vi "RTS Toggle Complete Buttons.vi"(7 "Delay":bool, 8 "Error In":errorcluster, 9 "Door Open Sequence:":T5, 10 "Times Up?":bool, 11 "Station 1-8 Data in in":T1 {"Station Slide"."Chamber 1-1"."Start Time" format="%<%X\n%x>T"; "Station Slide"."Chamber 1-1"."End Time" format="%<%X\n%x>T"; "Station Slide"."Time Count (s)" format="%.2f"; "Station Cab"."Chamber 1-1"."Start Time" format="%<%X\n%x>T"; "Station Cab"."Chamber 1-1"."End Time" format="%<%X\n%x>T"; "Station Cab"."Time Count (s)" format="%.2f"; "Station Freezer"."Chamber 1-1"."Start Time" format="%<%X\n%x>T"; "Station Freezer"."Chamber 1-1"."End Time" format="%<%X\n%x>T"; "Station Freezer"."Time Count (s)" format="%.2f"}) -> (0 "Error Out":errorcluster, 3 "Station 1-8 Data in out":T1 {"Station Slide"."Chamber 1-1"."Start Time" format="%<%X\n%x>T"; "Station Slide"."Chamber 1-1"."End Time" format="%<%X\n%x>T"; "Station Slide"."Time Count (s)" format="%.2f"; "Station Cab"."Chamber 1-1"."Start Time" format="%<%X\n%x>T"; "Station Cab"."Chamber 1-1"."End Time" format="%<%X\n%x>T"; "Station Cab"."Time Count (s)" format="%.2f"; "Station Freezer"."Chamber 1-1"."Start Time" format="%<%X\n%x>T"; "Station Freezer"."Chamber 1-1"."End Time" format="%<%X\n%x>T"; "Station Freezer"."Time Count (s)" format="%.2f"})   [LabVIEW 2016]
uses:
  Type Definitions/RTS Door Ops Sequence.ctl
  Type Definitions/RTS Station Relay Ops.ctl
  Type Definitions/RTS Door Opener Indicator.ctl
  Type Definitions/RTS Door Ops Client.ctl
  Type Definitions/RTS Door Opening Schedule.ctl
panel:
  # "Chamber Conditions:"
  # "Chamber Conditions:"
  # "Chamber Conditions:"
  # "Chamber Conditions:"
  # "Chamber Conditions:"
  # "Chamber Conditions:"
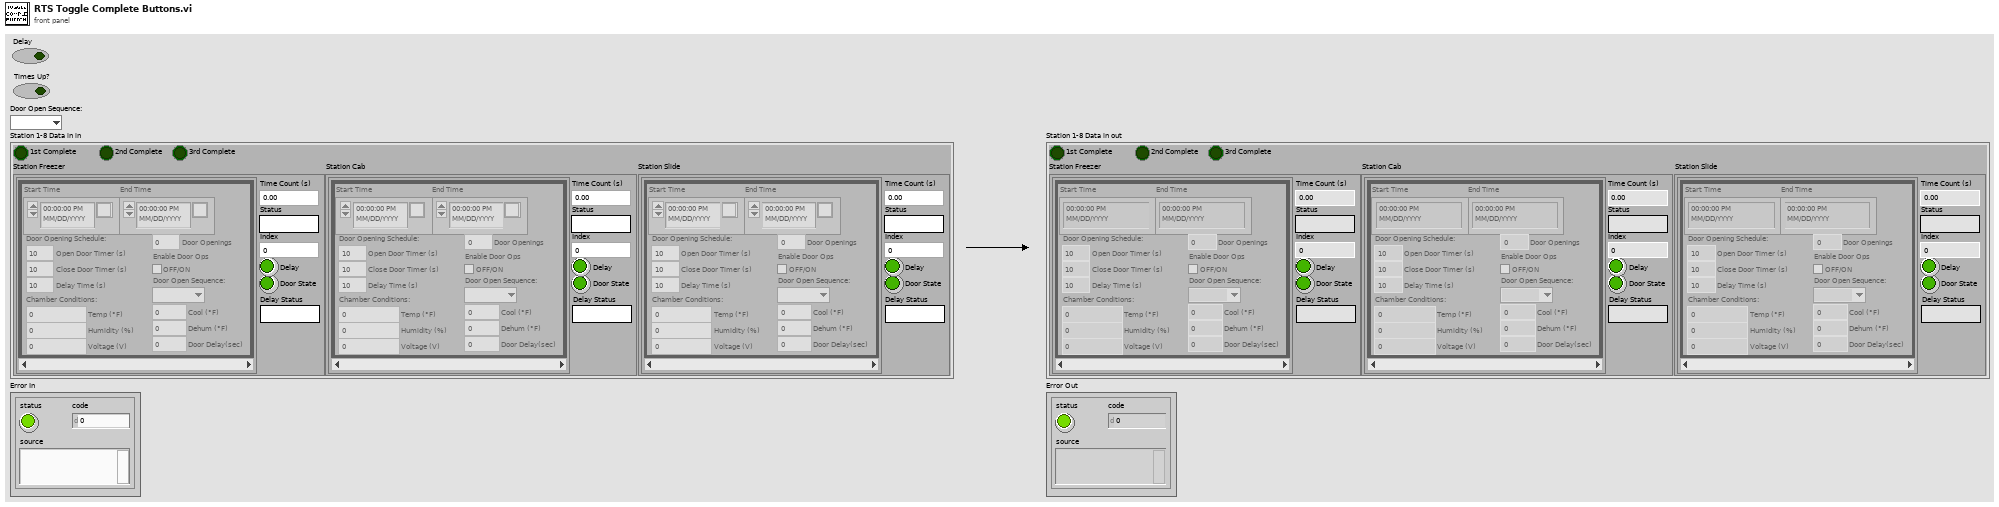
[diagram p1: front panel]
types:
  T1 = typedef "RTS Station Relay Ops.ctl" = cluster{"Station Freezer":T2, "Station Cab":T2, "Station Slide":T2, "1st Complete":bool, "2nd Complete":bool, "3rd Complete":bool}
  T2 = typedef "RTS Door Opener Indicator.ctl" = cluster{"Time Count (s)":dbl, "Status":string, "Door State":bool, "Delay":bool, "Chamber 1-1":T3[], "Index":i32, "Delay Status":string}
  T3 = typedef "RTS Door Ops Client.ctl" = cluster{"End Time":timestamp, "Start Time":timestamp, "Door Opening Schedule:":T4, "Enable Door Ops":bool, "Door Openings":u32, "Temp (°F)":dbl, "Humidity (%)":dbl, "Voltage (V)":dbl, "Door Open Sequence:":T5, "Door Delay(sec)":dbl, "Dehum (°F)":dbl, "Cool (°F)":dbl}
  T4 = typedef "RTS Door Opening Schedule.ctl" = cluster{"Open Door Timer (s)":dbl, "Delay Time (s)":dbl, "Close Door Timer (s)":dbl}
  T5 = typedef "RTS Door Ops Sequence.ctl" = enum16{"", "1st", "2nd", "3rd"}
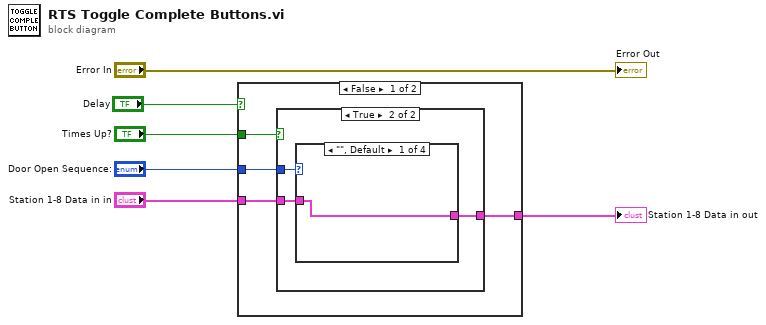
[diagram p0: block diagram]
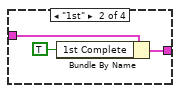
[diagram p3: hidden frame]
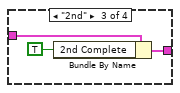
[diagram p4: hidden frame]
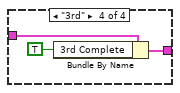
[diagram p5: hidden frame]
diagram:
  n1 = case shown="False" "Delay" {
    tunnel: "Door Open Sequence:" -> [w10 _]
    tunnel: "Station 1-8 Data in in" -> [w9 w25]
    tunnel: "Times Up?" -> [w8 _]
    tunnel: [w7 w25] -> w3
    frame False {
      n2 = case shown="True" w8 {
        tunnel: w9 -> [w11 w13]
        tunnel: [w11 w14] -> w7
        tunnel: w10 -> [_ w12]
        frame False {
        }
        frame True {
          n3 = case shown="\"\", Default" w12 {
            tunnel: [w15 w16 w21 w22] -> w14
            tunnel: w13 -> [w15 w17 w20 w23]
            frame "", Default {
            }
            frame "1st" {
              n4 = Bundle By Name(cluster=w17, "1st Complete"=TRUE) -> (w16:T1)
            }
            frame "2nd" {
              n5 = Bundle By Name(cluster=w20, "2nd Complete"=TRUE) -> (w21:T1)
            }
            frame "3rd" {
              n6 = Bundle By Name(cluster=w23, "3rd Complete"=TRUE) -> (w22:T1)
            }
          }
        }
      }
    }
    frame True {
    }
  }
  "Station 1-8 Data in out" <- w3
  "Error Out" <- "Error In"
